vi "PixelToMicronConversion (SubVI).vi"(9 "Template Image":path=path "C:/Users/Sciolla Lab/Pictures/10StripsGeometricTemplate.png", 11 "Path to images to calculate with":path=path "C:/Users/Sciolla Lab/Desktop/MoreCornersNames/image_44_30_1_01.png") -> (1 "Average microns/pixel":ext, 3 "standard dev on microns/pixel":ext)   [LabVIEW 2016]
doc: "This example shows how to use the geometric matching tools in NI Vision.\n\nGeometric matching is the technique used to quickly locate known reference or fiducial patterns in an image using edge information. Geometric matching is the key to many applications. Geometric matching can provide your application with information about the presence or absence, number, and location of the model within an image.\n\nAn important step in geometric matching is training the template. A specialized geometric training interface is provided for simple training with advanced features. This utility can be found at Start»Programs»National Instruments»Vision, or from Vision Assistant or Vision Builder for Automated Inspection."
uses:
  <vilib>/vision/Pattern Matching.llb/IMAQ Match Range Setting.ctl
  <vilib>/vision/NI_Vision_Development_Module.lvlib
  <vilib>/Analysis/NI_AALBase.lvlib
panel:
  in  "Range Settings":T1[](array[typedef]) {"Max" format="%.2f"; "Min" format="%.2f"; "Match Constraints" items=["Rotation Angle (degrees)", "Scale Factor (%)", "Occlusion (%)"]}
  in  "Naming Convention":string="image_442_-22_00.png"
  out "Results":string[][](table)
  in  "Minimum Score":sgl=800.0
  in  "Number of Matches":i32=4
  out "Template":T2(plugin-control)
  out "Image":T2(plugin-control)
  # "Overview: This takes a set of images which include strips and a template (given) and finds the pixel to micron ratio average and standard deviation across images. \nRequirements: NI Vision Development Module\nInstructions: Select an image in your path and naming convention of images.  Run to find microns/pixel and standard deviation."
  # "Range"
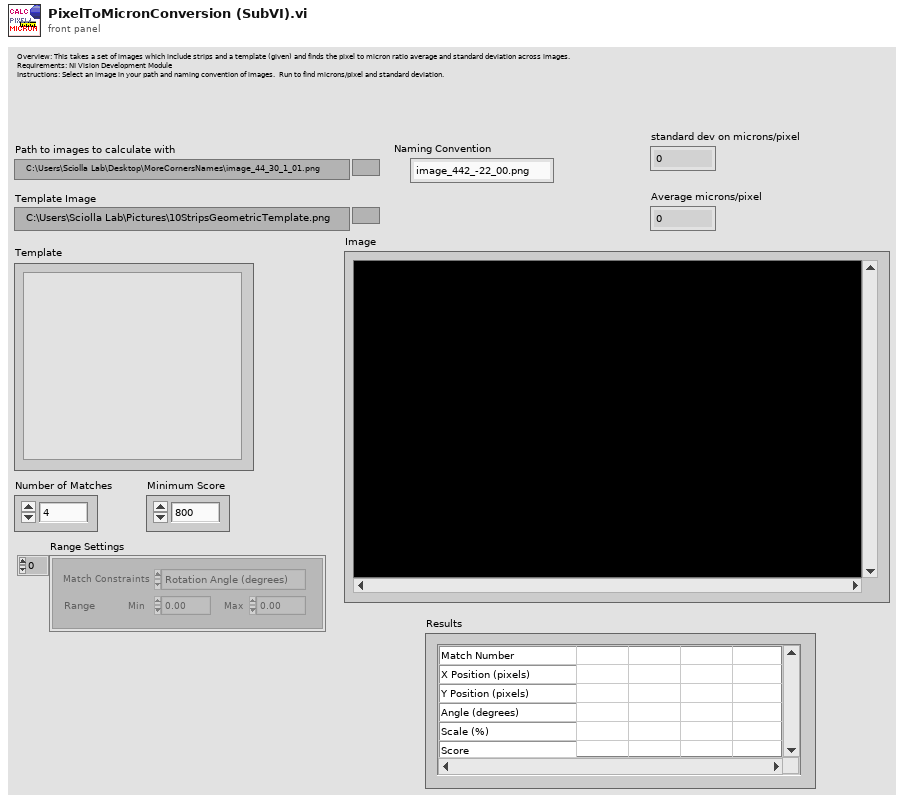
[diagram p1: front panel]
types:
  T1 = typedef "IMAQ Match Range Setting.ctl" = cluster{"Match Constraints":u32, "Min":dbl, "Max":dbl}
  T2 = typedef "IMAQ Image.ctl" = refnum<image>
  T3 = typedef "Image Type" = u32
  T4 = cluster{"Rotation":bool, "Scale":bool, "Occlusion":bool, "Reserved":bool, "Reserved":bool, "Reserved":bool}
  T5 = typedef "IMAQ GM Match Report.ctl" = cluster{"Position":cluster{"x":sgl, "y":sgl}, "Angle":sgl, "Scale":sgl, "Score":sgl, "Bounding Box":cluster{"x":sgl, "y":sgl}[], "Contrast Reversed":bool, "Occlusion %":sgl, "Template Target Curve Score":sgl, "Target Template Curve Score":sgl, "Correlation Score":sgl}
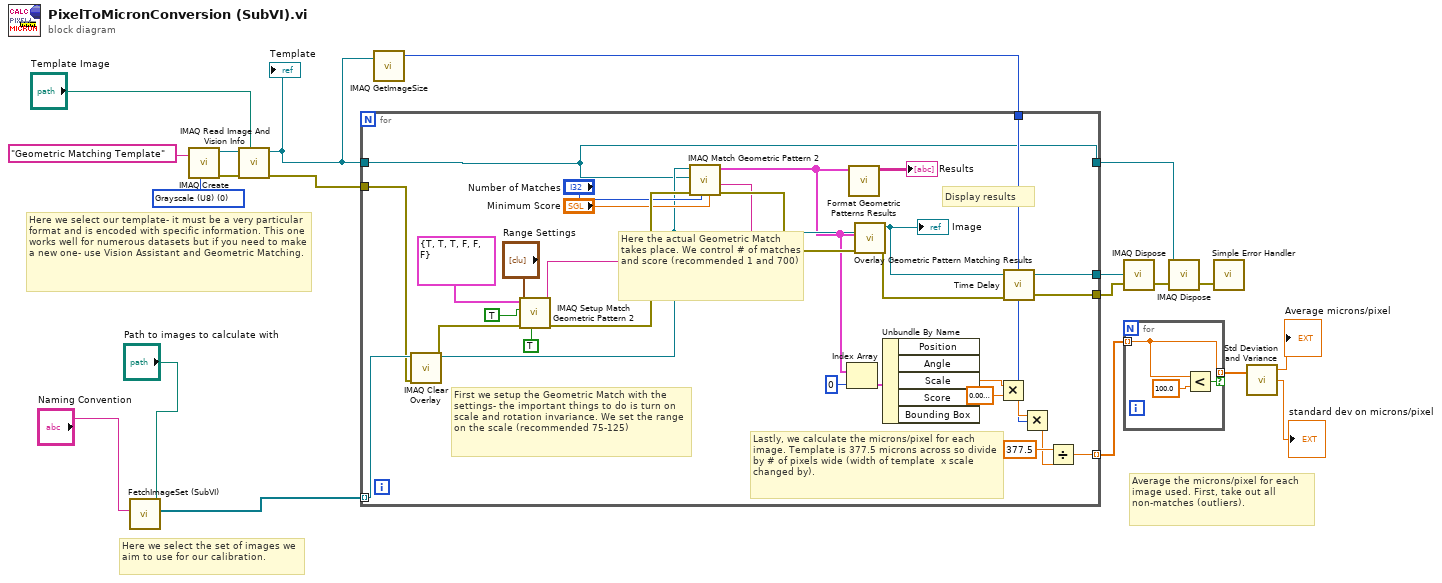
[diagram p0: block diagram]
diagram:
  w17 = T3 0 items=["Grayscale (U8)", "Grayscale (I16)", "Grayscale (SGL)", "Complex (CSG)", "RGB (U32)", "HSL (U32)", "RGB (U64)"] ("Image Type")
  # "Average the microns/pixel for each image used. First, take out all non-matches (outliers)."
  # "Here we select the set of images we aim to use for our calibration."
  # "Here we select our template- it must be a very particular format and is encoded with specific information. This one works well for numerous datasets but if you need to make a new one- use Vision Assistant and Geometric Matching."
  n1 = call "FetchImageSet (SubVI).vi"("Naming Convention"="Naming Convention", "Images Directory"="Path to images to calculate with") -> ("Image Array"=w6:T2[])  [unwired: 7 in, 2 out]
  n2 = call "IMAQ Create"("Image Name"="Geometric Matching Template", "Image Type"=w17) -> ("New Image"=w18:T2, "error out"=w19:errorcluster)  [unwired: 2 in, 1 out]
  n3 = call "IMAQ Read Image And Vision Info"("File Path"="Template Image", "error in (no error)"=w19, "Image"=w18) -> ("error out"=w11:errorcluster, "Image Out"=w9:T2)  [unwired: 1 in, 6 out]
  "Template" <- w9
  n4 = call "IMAQ GetImageSize"("Image"=w9) -> ("X Resolution"=w8:i32)  [unwired: 3 in, 2 out]
  n5 = for {
    tunnel: [w48] -> w20
    tunnel: w9 -> [w25]
    tunnel: [w38] -> w15
    tunnel: [w25] -> w14
    tunnel: w11 -> [w21]
    tunnel: [w29] -> w1 mode=indexing
    tunnel: w8 -> [w28]
    tunnel: w6 -> [w27] mode=indexing
    # "Display results"
    # "Here the actual Geometric Match takes place. We control # of matches and score (recommended 1 and 700)"
    # "First we setup the Geometric Match with the settings- the important things to do is turn on scale and rotation invariance. We set the range on the scale (recommended 75-125)"
    # "Lastly, we calculate the microns/pixel for each image. Template is 377.5 microns across so divide by # of pixels wide (width of template  x scale changed by)."
    n6 = call "IMAQ Clear Overlay"("error in (no error)"=w21, "Image"=w27) -> ("error out"=w42:errorcluster, "Image Out"=w40:T2)  [unwired: 1 in, 7 out]
    n7 = call "IMAQ Setup Match Geometric Pattern 2"("Use Learn Curve Parameters"=TRUE, "error in (no error)"=w42, "Range Settings"="Range Settings", "Subpixel Accuracy"=TRUE, "Match Mode"=T4 {"Rotation"=TRUE, "Scale"=TRUE, "Occlusion"=TRUE, "Reserved"=FALSE, "Reserved"=FALSE, "Reserved"=FALSE}) -> ("error out"=w47:errorcluster, "Match Geometric Pattern 2 Setup Data"=w22:string)  [unwired: 1 in, 4 out]
    n8 = call "IMAQ Match Geometric Pattern 2"("Minimum Match Score"="Minimum Score", "Number of Matches Requested"="Number of Matches", "error in (no error)"=w47, "Match Geometric Pattern 2 Setup Data"=w22, "Template Image"=w25, "Image"=w40) -> ("error out"=w43:errorcluster, "Matches (pixel)"=w37:T5[])  [unwired: 1 in, 3 out]
    n9 = Index Array(array=w37, index=0) -> (element=w35:T5)
    n10 = call "Format Geometric Patterns Results.vi"("Matches"=w37) -> ("Text Results"=→"Results":string[][])  [unwired: 9 in, 1 out]
    n11 = call "Overlay Geometric Pattern Matching Results.vi"("error in"=w43, "Matches"=w37, "Image"=w40) -> ("error out"=w41:errorcluster, "Image Out"=w38:T2)  [unwired: 2 in, 5 out]
    "Image" <- w38
    n12 = Unbundle By Name(w35) -> ("Scale"=w34:sgl)  [unwired: 4 out]
    n13 = Multiply(x=w34, y=sgl 0.01) -> (x*y=w32:sgl)
    n14 = call "Time Delay"("error in (no error)"=w41) -> ("error out"=w48:errorcluster)  [unwired: 10 in]
    n15 = Multiply(x=w32, y=w28) -> (x*y=w30:sgl)
    n16 = Divide(x=377.5, y=w30) -> (x/y=w29:dbl)
  }
  n17 = call "IMAQ Dispose"("Image"=w15, "error in (no error)"=w20) -> ("error out"=w13:errorcluster)  [unwired: 1 in, 3 out]
  n18 = for {
    tunnel: w1 -> [w50] mode=indexing
    tunnel: [w50] -> w2 mode=indexing if=w49
    n19 = Less?(x=w50, y=100.0) -> (x < y?=w49:bool)
  }
  n20 = call "IMAQ Dispose"("Image"=w14, "error in (no error)"=w13) -> ("error out"=w12:errorcluster)  [unwired: 1 in, 3 out]
  n21 = call <vilib>:"Simple Error Handler.vi"("error in (no error)"=w12) -> ()  [unwired: 4 in, 5 out]
  n22 = call <vilib>:"Std Deviation and Variance.vi"("X"=w2) -> ("mean"=→"Average microns/pixel":dbl, "standard deviation"=→"standard dev on microns/pixel":dbl)  [unwired: 1 in, 1 out]
